vi "JTrkMinimalTest.vi"   [LabVIEW 2011]
uses:
  JelmersTracker.llb/TrackerDLL.vi
types:
  T1 = typedef "TrackerInstance.ctl" = cluster{"Tracker Pointer":u64, "Image size":cluster{"width":u32, "height":u32}}
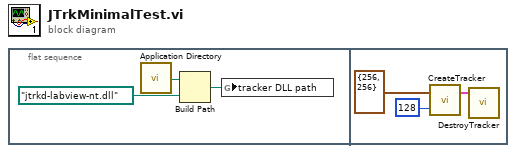
[diagram p0: block diagram]
diagram:
  n1 = flat-sequence {
    frame #0 {
      n2 = call <vilib>:"Application Directory.vi"() -> ("Application Directory"=w2:path)
      n3 = Build Path(base path=w2, name or relative path=path "jtrkd-labview-nt.dll") -> (appended path=w1:path)
      n4 = global write "TrackerDLL.vi" "tracker DLL path"(w1) -> ()
    }
    frame #1 {
      n5 = call "CreateTracker.vi"("XCorWindow"=u32 128, "Image size"=cluster{"width":u32, "height":u32} {"width"=256, "height"=256}) -> ("tracker"=w4:T1)  [unwired: 1 in]
      n6 = call "DestroyTracker.vi"("tracker instance"=w4) -> ()  [unwired: 5 in]
    }
  }
